vi "measure_max-power-stabilisation.vi"(0 "User Name":string, 1 "Cell details cluster":T2={"Cell Position"=16, "Cell Label"="", "Pixel to measure"=0, "Area (cm^2)"=0.126, "Variable"="", "Variable value"="", "Scan settings in queue"=0, "Light or dark"="", "Measurement Type"=""} {"Pixel to measure" items=["All", "1", "2", "3", "4", "5", "6", "7", "8"]}, 3 "Date array":string[](array[string]), 5 "Experiment Title":string, 9 "File path of JV log":path, 11 "Intensity (no. of suns)":string, 12 "Scan settings":T1={"J-V scan"=TRUE, "Start voltage (V)"=0.0, "End voltage (V)"=0.0, "Step voltage (V)"=1.4, "Scan both directions"=TRUE, "Inverted device structure"=FALSE, "Measurement delay (ms)"=10.0, "Measurement speed"=0, "Scan rate (V/s)"=0.0, "Stabilisation time (s)"=0.0, "Stabilisation mode"=0, "Stabilisation value (V or A) "=1.0, "Illumination"=0, "Stabilisation in the dark?"=FALSE, "Repeat light scans"=FALSE, "No. of repeat scans"=0.0, "Only repeat for best pixel"=1, "J-t scan"=FALSE, "J-t best pixel only"=7, "J-t start voltage (V)"=0.0, "J-t end voltage (V)"=1.4, "J-t step voltage (V)"=0.01, "Step time (s)"=0.7, "J-t scan both directions"=TRUE, "J-t inverted device structure"=FALSE, "J-t settling delay (s)"=0.0, "J-t measurement speed"=0, "J-t illumination"=2, "Max. power stabilisation"=FALSE, "Max power best pixel only"=1, "Max. power point tracker"=FALSE, "Vmp from J-V scan"=FALSE, "Max P stab. Specific voltage"=FALSE, "Vmp (V)"=1.0, "Stabilisation time step (s)"=1.0, "Total stabilisation time (s)"=100.0} {"J-t settling delay (s)" min=10.0; "J-t illumination" items=["Light only", "Dark only", "Light then dark", "Dark then light"]; "Measurement speed" items=["Fast", "Normal", "High accuracy"]; "Illumination" items=["Light only", "Dark only", "Light then dark", "Dark then light"]; "Only repeat for best pixel" items=["only for best pixel", "for best 2 pixels", "for best 3 pixels", "for best 4 pixels", "for best 5 pixels", "for best 6 pixels", "for best 7 pixels", "for all pixels"]; "No. of repeat scans" min=1.0 step=1.0; "Max power best pixel only" items=["only the best pixel", "the best 2 pixels", "the best 3 pixels", "the best 4 pixels", "the best 5 pixels", "the best 6 pixels", "the best 7 pixels", "all pixels"]; "J-t best pixel only" items=["only the best pixel", "the best 2 pixels", "the best 3 pixels", "the best 4 pixels", "the best 5 pixels", "the best 6 pixels", "the best 7 pixels", "all pixels"]; "J-t measurement speed" items=["Fast", "Normal", "High Accuracy"]; "Stabilisation mode" items=["V", "I"]; "Measurement delay (ms)" min=10.0}, 13 "VISA resource name":refnum<visa-resource-name>="GPIB1::24::INSTR", 14 "Skip pixel?":bool) -> (4 "Jt Curve":cluster{"Y":dbl[], "Y":dbl[]}[](graph) caption="JV Curve")   [LabVIEW 2016]
uses:
  TypeDefs/scan_settings.ctl
  <vilib>/Utility/file.llb/Read Delimited Spreadsheet (DBL).vi
panel:
  out "VISA resource name 2":refnum<visa-resource-name>="GPIB1::24::INSTR"
  out "File path for Jt image":path
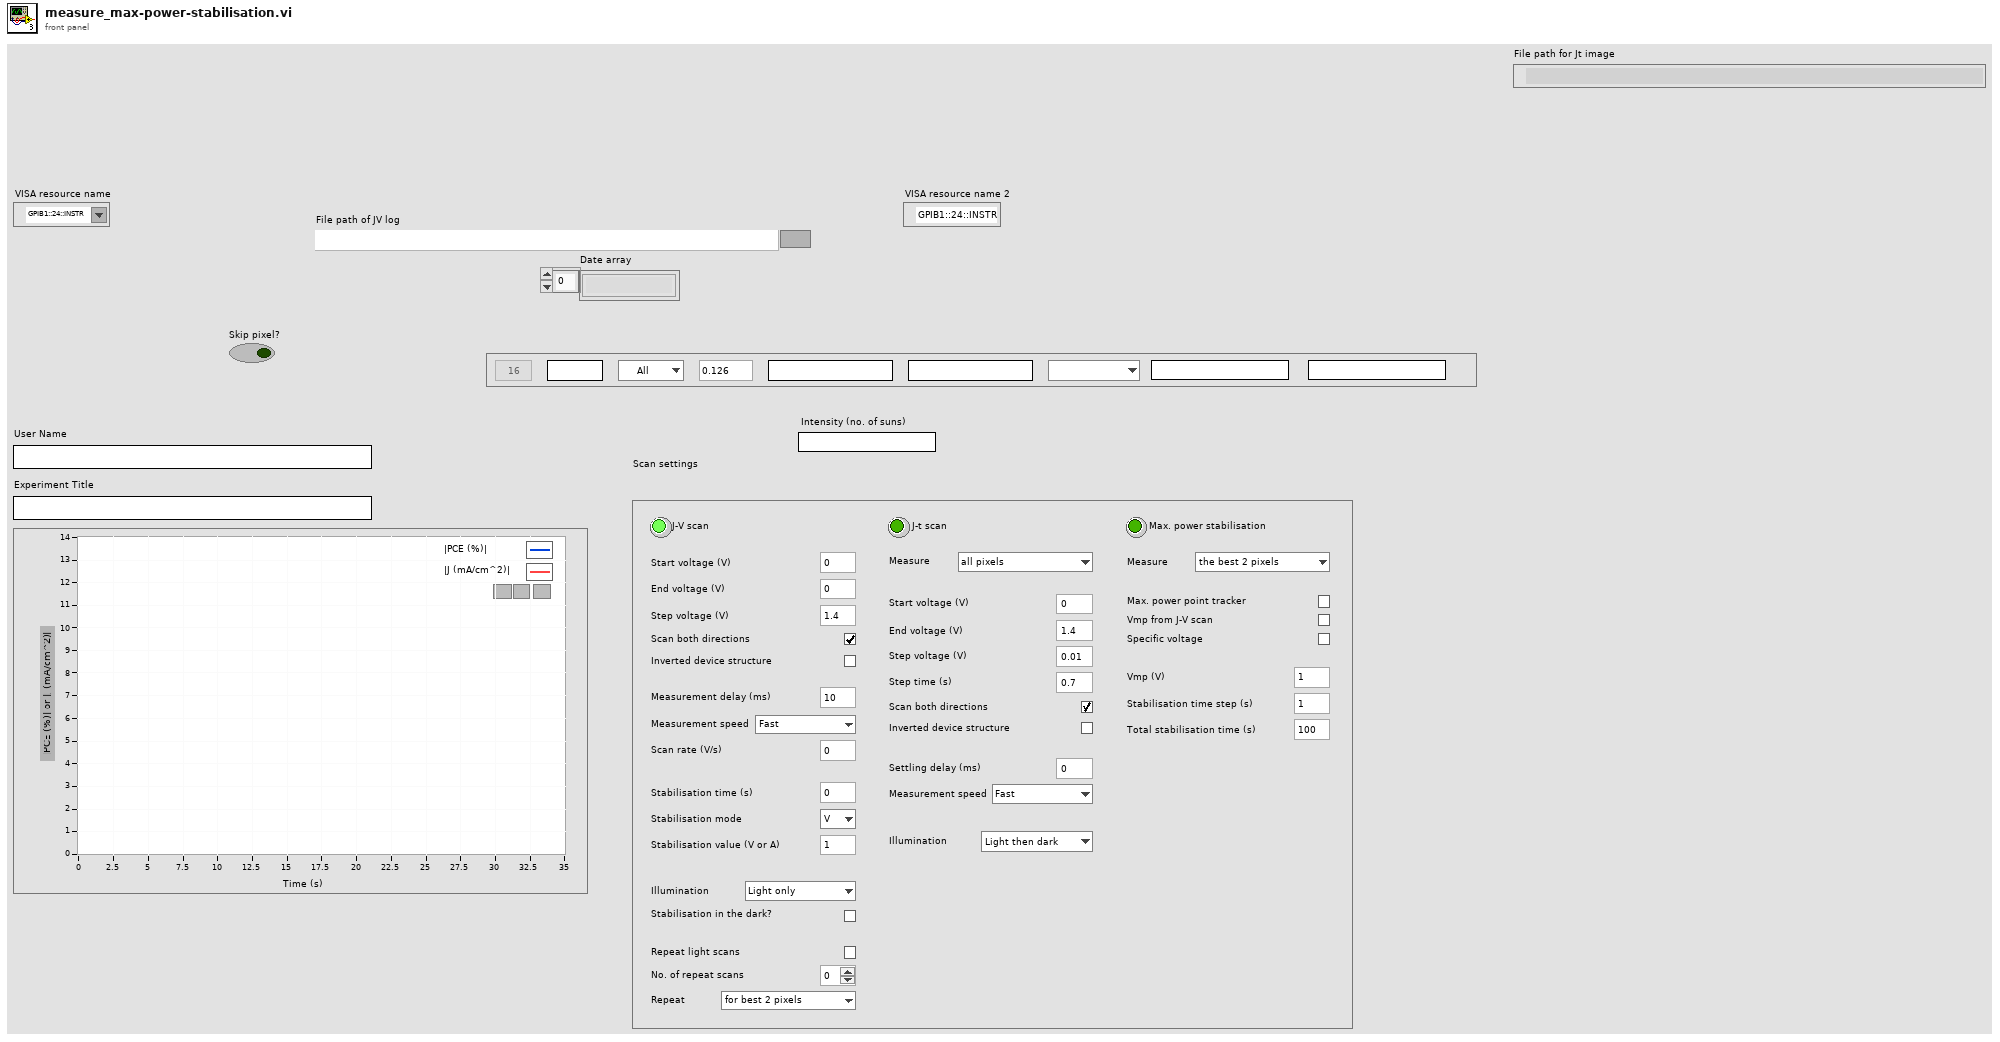
[diagram p1: front panel]
types:
  T1 = typedef "scan_settings.ctl" = cluster{"J-V scan":bool, "Start voltage (V)":dbl, "End voltage (V)":dbl, "Step voltage (V)":dbl, "Scan both directions":bool, "Inverted device structure":bool, "Measurement delay (ms)":dbl, "Measurement speed":u8, "Scan rate (V/s)":dbl, "Stabilisation time (s)":dbl, "Stabilisation mode":u16, "Stabilisation value (V or A) ":dbl, "Illumination":u16, "Stabilisation in the dark?":bool, "Repeat light scans":bool, "No. of repeat scans":dbl, "Only repeat for best pixel":u16, "J-t scan":bool, "J-t best pixel only":u16, "J-t start voltage (V)":dbl, "J-t end voltage (V)":dbl, "J-t step voltage (V)":dbl, "Step time (s)":dbl, "J-t scan both directions":bool, "J-t inverted device structure":bool, "J-t settling delay (s)":dbl, "J-t measurement speed":u16, "J-t illumination":u16, "Max. power stabilisation":bool, "Max power best pixel only":u16, "Max. power point tracker":bool, "Vmp from J-V scan":bool, "Max P stab. Specific voltage":bool, "Vmp (V)":dbl, "Stabilisation time step (s)":dbl, "Total stabilisation time (s)":dbl}
  T2 = cluster{"Cell Position":i32, "Cell Label":string, "Pixel to measure":u16, "Area (cm^2)":dbl, "Variable":string, "Variable value":string, "Scan settings in queue":u16, "Light or dark":string, "Measurement Type":string}
  T3 = typedef "imagedata.ctl" = cluster{"image type":i32, "image depth":i32, "image":u8[], "mask":u8[], "colors":u32[], "Rectangle":cluster{"left":i16, "top":i16, "right":i16, "bottom":i16}}
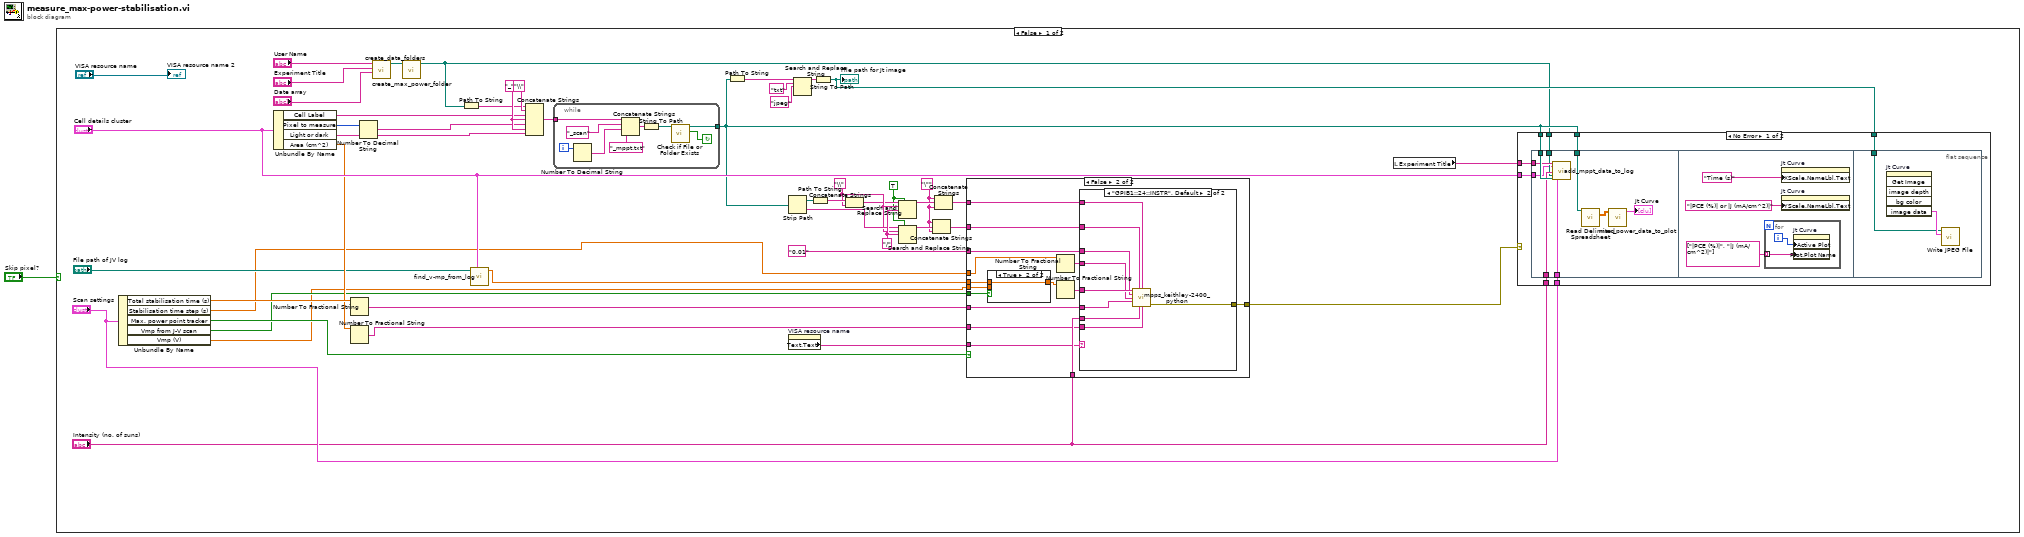
[diagram p0: block diagram]
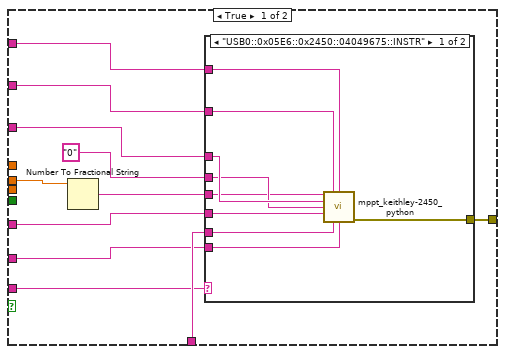
[diagram p2: hidden frame]
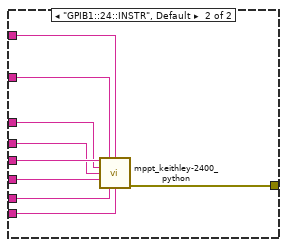
[diagram p3: hidden frame]
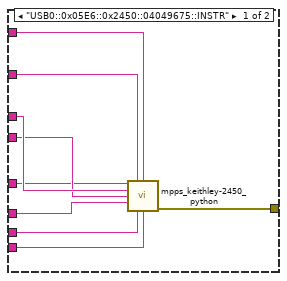
[diagram p5: hidden frame]
diagram:
  n1 = case shown="False" "Skip pixel?" {
    frame False {
      w21 = "\"" ("string")
      w12 = TRUE ("replace all? (F)")
      w32 = "/" ("search string")
      w20 = "\\" ("search string")
      w41 = "_"
      n2 = Unbundle By Name("Scan settings") -> ("Total stabilisation time (s)"=w48:dbl, "Stabilisation time step (s)"=w3:dbl, "Max. power point tracker"=w7:bool, "Vmp from J-V scan"=w6:bool, "Vmp (V)"=w4:dbl)
      n3 = Unbundle By Name("Cell details cluster") -> ("Cell Label"=w37:string, "Pixel to measure"=w38:u16, "Light or dark"=w35:string, "Area (cm^2)"=w29:dbl)
      n4 = Number To Fractional String(number=w29) -> (F-format string=w18:string)  [unwired: 3 in]
      n5 = Number To Fractional String(number=w48) -> (F-format string=w17:string)  [unwired: 3 in]
      n6 = Number To Decimal String(number=w38) -> (decimal integer string=w36:string)  [unwired: 1 in]
      n7 = call "create_data_folders.vi"("Date array"="Date array", "Experiment Indicator"="Experiment Title", "username"="User Name") -> ("Data Output Folder"=w42:path)  [unwired: 8 in]
      n8 = call "create_max_power_folder.vi"("Data Folder In"=w42) -> ("Data Output Folder"=w22:path)  [unwired: 10 in]
      n9 = Path To String(path=w22) -> (string=w33:string)
      n10 = call "find_v-mp_from_log.vi"("Cell details cluster in"="Cell details cluster", "File path of JV log"="File path of JV log") -> ("Vmp"=w5:dbl)  [unwired: 9 in]
      n11 = Concatenate Strings(w33, "\\", w37, w41, w36, w41, w35) -> (w40:string)
      n12 = while {
        tunnel: w40 -> [w147]
        tunnel: [w139] -> w24
        i -> [w145]
        stop <- w140 continue-if-true
        n13 = Number To Decimal String(number=w145) -> (decimal integer string=w144:string)  [unwired: 1 in]
        n14 = Concatenate Strings(w147, "_scan", w144, "_mppt.txt") -> (w141:string)
        n15 = String To Path(string=w141) -> (path=w142:path)
        n16 = call <vilib>:"Check if File or Folder Exists.vi"("path"=w142) -> ("file or folder exists?"=w140:bool, "dup path"=w139:path)  [unwired: 8 in, 1 out]
      }
      n17 = Path To String(path=w24) -> (string=w46:string)
      n18 = Strip Path(path=w24) -> (stripped path=w27:path, name=w28:string)
      n19 = property on="VISA resource name" class="VISAName"() -> ("Text.Text"=w11:string)  [unwired: 2 in, 2 out]
      n20 = Search and Replace String(input string=w46, search string="txt", replace string="jpeg") -> (result string=w43:string)  [unwired: 5 in, 3 out]
      n21 = Path To String(path=w27) -> (string=w26:string)
      n22 = String To Path(string=w43) -> (path=w30:path)
      "File path for Jt image" <- w30
      n23 = Concatenate Strings(w26, w20) -> (w13:string)
      n24 = Search and Replace String(replace all?=w12, input string=w28, search string=w20, replace string=w32) -> (result string=w31:string)  [unwired: 4 in, 3 out]
      n25 = Search and Replace String(replace all?=w12, input string=w13, search string=w20, replace string=w32) -> (result string=w34:string)  [unwired: 4 in, 3 out]
      n26 = Concatenate Strings(w21, w31, w21) -> (w15:string)
      n27 = Concatenate Strings(w21, w34, w21) -> (w16:string)
      n28 = case shown="False" w7 {
        tunnel: "Intensity (no. of suns)" -> [w61 w94]
        tunnel: [w60 w93] -> w19
        tunnel: w18 -> [w59 w92]
        tunnel: w17 -> [w58 w91]
        tunnel: w16 -> [w57 w90]
        tunnel: w15 -> [w56 w89]
        tunnel: "0.01" ("search string") -> [w55 w88]
        tunnel: w11 -> [w54 w87]
        tunnel: w6 -> [_ w85]
        tunnel: w5 -> [w53 w83]
        tunnel: w4 -> [_ w82]
        tunnel: w3 -> [_ w80]
        frame True {
          n29 = Number To Fractional String(number=w53) -> (F-format string=w52:string)  [unwired: 3 in]
          n30 = case shown="\"USB0::0x05E6::0x2450::04049675::INSTR\"" w54 {
            tunnel: [w70 w79] -> w60
            tunnel: w61 -> [w63 w78]
            tunnel: w59 -> [w62 w77]
            tunnel: w58 -> [w64 w76]
            tunnel: w52 -> [w65 w75]
            tunnel: w57 -> [w69 w74]
            tunnel: w56 -> [w68 w73]
            tunnel: w55 -> [w67 w72]
            tunnel: "0" ("search string") -> [w66 w71]
            frame "USB0::0x05E6::0x2450::04049675::INSTR" {
              n31 = call "mppt_keithley-2450_python.vi"("start voltage (V)"=w65, "file name"=w68, "folder path"=w69, "nplc"=w67, "settling delay (s)"=w66, "total tracking time (s)"=w64, "illumination intensity (suns equiv.)"=w63, "area (cm^2)"=w62) -> ("error out"=w70:errorcluster)  [unwired: 7 in]
            }
            frame "GPIB1::24::INSTR", Default {
              n32 = call "mppt_keithley-2400_python.vi"("start voltage (V)"=w75, "file name"=w73, "folder path"=w74, "nplc"=w72, "settling delay (s)"=w71, "total tracking time (s)"=w76, "illumination intensity (suns equiv.)"=w78, "area (cm^2)"=w77) -> ("error out"=w79:errorcluster)  [unwired: 7 in]
            }
          }
        }
        frame False {
          n33 = case shown="True" w85 {
            tunnel: [w95 w96] -> w84
            tunnel: w83 -> [_ w96]
            tunnel: w82 -> [w95 _]
            frame False {
            }
            frame True {
            }
          }
          n34 = Number To Fractional String(number=w80) -> (F-format string=w81:string)  [unwired: 3 in]
          n35 = Number To Fractional String(number=w84) -> (F-format string=w86:string)  [unwired: 3 in]
          n36 = case shown="\"GPIB1::24::INSTR\", Default" w87 {
            tunnel: [w105 w114] -> w93
            tunnel: w94 -> [w98 w113]
            tunnel: w92 -> [w97 w112]
            tunnel: w91 -> [w99 w111]
            tunnel: w86 -> [w100 w110]
            tunnel: w90 -> [w104 w109]
            tunnel: w89 -> [w103 w108]
            tunnel: w88 -> [w102 w107]
            tunnel: w81 -> [w101 w106]
            frame "USB0::0x05E6::0x2450::04049675::INSTR" {
              n37 = call "mpps_keithley-2450_python.vi"("start voltage (V)"=w100, "file name"=w103, "folder path"=w104, "nplc"=w102, "settling delay (s)"=w101, "total tracking time (s)"=w99, "illumination intensity (suns equiv.)"=w98, "area (cm^2)"=w97) -> ("error out"=w105:errorcluster)  [unwired: 7 in]
            }
            frame "GPIB1::24::INSTR", Default {
              n38 = call "mpps_keithley-2400_python.vi"("start voltage (V)"=w110, "file name"=w108, "folder path"=w109, "nplc"=w107, "settling delay (s)"=w106, "total tracking time (s)"=w111, "illumination intensity (suns equiv.)"=w113, "area (cm^2)"=w112) -> ("error out"=w114:errorcluster)  [unwired: 7 in]
            }
          }
        }
      }
      n39 = local read "Experiment Title"() -> (w23:string)
      n40 = case shown="No Error" w19 {
        tunnel: w24 -> [w122 _]
        tunnel: w30 -> [w121 _]
        tunnel: "Scan settings" -> [w120 _]
        tunnel: w24 -> [w119 _]
        tunnel: "Intensity (no. of suns)" -> [w118 _]
        tunnel: w23 -> [w117 _]
        tunnel: w22 -> [w116 _]
        tunnel: "Cell details cluster" -> [w115 _]
        frame No Error {
          n41 = flat-sequence {
            tunnel: w122 -> [w131]
            tunnel: w120 -> [w129]
            tunnel: w119 -> [w128]
            tunnel: w118 -> [w127]
            tunnel: w117 -> [w126]
            tunnel: w116 -> [w125]
            tunnel: w115 -> [w124]
            tunnel: w121 -> [w137]
            frame #0 {
              n42 = call "add_mppt_data_to_log.vi"("Experiment Indicator"=w126, "Cell details cluster"=w124, "Intensity (no. of suns)"=w127, "mppt folder path"=w125, "mppt file path"=w128, "Scan settings"=w129) -> ()  [unwired: 12 in, 2 out]
              n43 = call-poly <vilib>:"Read Delimited Spreadsheet.vi"("file path (dialog if empty)"=w131) -> ("all rows"=w130:dbl[][])  [unwired: 9 in, 5 out]
              n44 = call "max_power_data_to_plot.vi"("Data Array"=w130) -> ("JV Curve"=→"Jt Curve":cluster{"Y":dbl[], "Y":dbl[]}[])  [unwired: 10 in]
            }
            frame #1 {
              n45 = for {
                tunnel: string[] ["|PCE (%)|", "|J (mA/cm^2)|"] ("Measurement queue") -> [w135] mode=indexing
                i -> [w136]
                n46 = property on="Jt Curve" class="XYGraph (strict)"("Active Plot"=w136, "Plot.Plot Name"=w135) -> ()  [unwired: 2 in, 2 out]
              }
              n47 = property on="Jt Curve" class="XYGraph (strict)"("XScale.NameLbl.Text"="Time (s)" ("Y Scale.Name Label.Text")) -> ()  [unwired: 2 in, 2 out]
              n48 = property on="Jt Curve" class="XYGraph (strict)"("YScale.NameLbl.Text"="|PCE (%)| or |J (mA/cm^2)|" ("Y Scale.Name Label.Text")) -> ()  [unwired: 2 in, 2 out]
            }
            frame #2 {
              n49 = invoke on="Jt Curve" class="XYGraph (strict)" method="Get Image"() -> ("image data"=w138:T3)  [unwired: 6 in, 5 out]
              n50 = call <vilib>:"Write JPEG File.vi"("image data"=w138, "path to JPEG file"=w137) -> ()  [unwired: 8 in, 2 out]
            }
          }
        }
        frame Error {
        }
      }
      "VISA resource name 2" <- "VISA resource name"
    }
    frame True {
    }
  }
